vi "PC_Main3.vi"() -> ()   [LabVIEW 2017]
uses:
  <vilib>/userdefined/High Color/IMAQdx.ctl
  pc_states.ctl
  pc_data.ctl
  <vilib>/vision/Image Controls.llb/IMAQ Image.ctl
  new_coordinate.ctl
  xy_motion_graphs.ctl
  <vilib>/vision/driver/NI_Vision_Acquisition_Software.lvlib
  <vilib>/vision/NI_Vision_Development_Module.lvlib
panel:
  out "Kicker Angle":dbl caption="Numeric" format="%#.1f°"
  out "Puck Y Post":dbl
  out "Puck X Post":sgl
  out "start time":timestamp
  out "Shot Count":i16 caption="Numeric"
  out "Theta  Angle":dbl caption="Numeric" format="%#_g°"
  out "Kicker Power":dbl caption="Numeric" format="%#.1g%%"
  in  "Config Input":T1
  out "Config Output":T3
  out "Elapsed Time (s)":dbl caption="Numeric" format="%#.1p"
  out "Y Axis":dbl[][](graph) caption="Waveform Chart"
  out "X Axis":dbl[][](graph) caption="Waveform Chart"
  in  "Bounce/Straight":bool
  in  "Live Feed":bool caption="Reset"
  in  "Start":bool
  in  "Filpped":bool
  out "Live Image":T4(plugin-control)
  in  "Config":bool
  out "Snapshot Image":T4(plugin-control)
  in  "Stop":bool
  # "Table Football"
  # "UI Elements by JKI"
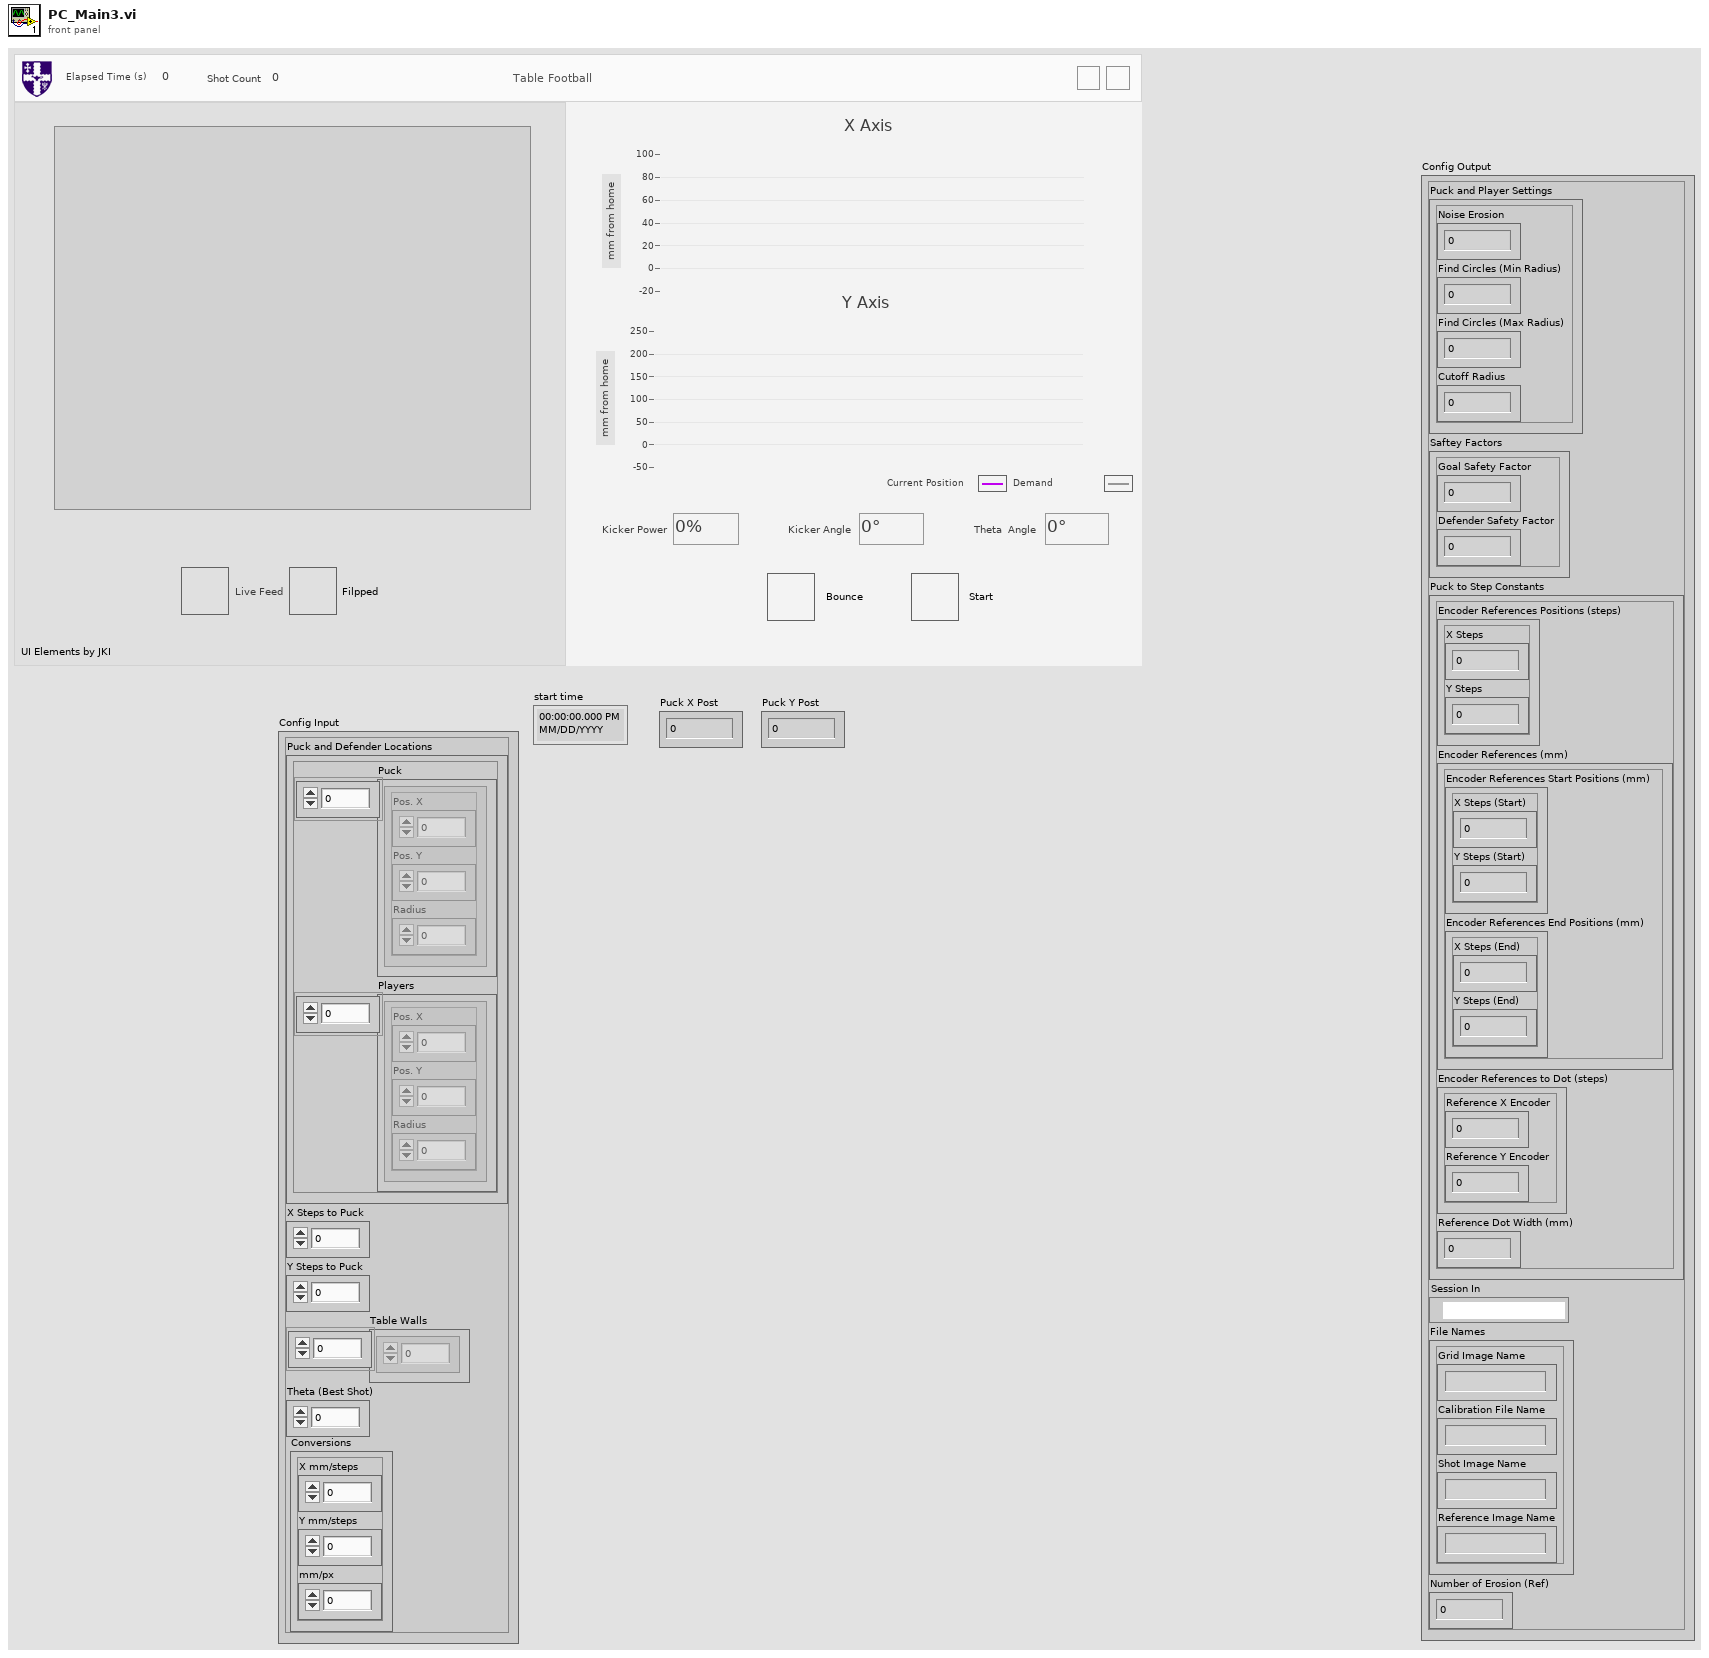
[diagram p1: front panel]
types:
  T1 = cluster{"Puck and Defender Locations":cluster{"Puck":cluster{"Pos. X":i32, "Pos. Y":i32, "Radius":i32}[], "Players":cluster{"Pos. X":i32, "Pos. Y":i32, "Radius":i32}[]}, "X Steps to Puck":dbl, "Y Steps to Puck":dbl, "Table Walls":sgl[], "Theta (Best Shot)":dbl, "Conversions":cluster{"X mm/steps":dbl, "Y mm/steps":dbl, "mm/px":dbl}}
  T2 = typedef "IMAQdx.ctl" = refnum<k21>
  T3 = cluster{"Puck and Player Settings":cluster{"Noise Erosion":i32, "Find Circles (Min Radius)":sgl, "Find Circles (Max Radius)":sgl, "Cutoff Radius  ":sgl}, "Saftey Factors":cluster{"Goal Safety Factor":dbl, "Defender Safety Factor":dbl}, "Puck to Step Constants":cluster{"Encoder References Positions (steps)":cluster{"X Steps":dbl, "Y Steps":dbl}, "Encoder References (mm)":cluster{"Encoder References Start Positions (mm)":cluster{"X Steps (Start)":dbl, "Y Steps (Start)":dbl}, "Encoder References End Positions (mm)":cluster{"X Steps (End)":dbl, "Y Steps (End)":dbl}}, "Encoder References to Dot (steps)":cluster{"Reference X Encoder":dbl, "Reference Y Encoder":dbl}, "Reference Dot Width (mm)":dbl}, "Session In":T2, "File Names":cluster{"Grid Image Name":string, "Calibration File Name":string, "Shot Image Name":string, "Reference Image Name":string}, "Number of Erosion (Ref)":i32}
  T4 = typedef "IMAQ Image.ctl" = refnum<image>
  T5 = typedef "pc_data.ctl" = cluster{"Camera Image":T4, "Reference Dimentions Out":cluster{"X":dbl, "Y":dbl, "Width":dbl}, "Table Walls":sgl[], "Player & Puck Locations":cluster{"Puck":cluster{"Pos. X":i32, "Pos. Y":i32, "Radius":i32}[], "Players":cluster{"Pos. X":i32, "Pos. Y":i32, "Radius":i32}[]}, "Theta (Best Shot)":dbl, "X Steps to Puck":dbl, "Y Steps to Puck":dbl, "Conversions":cluster{dbl, dbl, dbl}, "Shot Coordinate Template":cluster{cluster{"Straight Goal X":sgl, "Straight Goal Y":dbl}, cluster{"Bounce Wall X":dbl, "Bounce Wall Y":sgl}, cluster{"Bounce Goal X":sgl, "Bounce Goal Y":dbl}}, "Shot Power":dbl}
  T6 = typedef "Image Type" = u32
  T7 = typedef "pc_states.ctl" = cluster{enum16{"Stop", "Startup", "New Calibration Image", "Create Calibration File", "New Reference Image", "Apply Calibration (Ref)", "Find Reference Dot", "New Table Image", "Apply Calibration (Tab)", "Find Pucks, Players & Corners", "Calculate Shot Trajectories", "Calculate Puck to Steps", "Clear Best Shot Overlay", "Send Coordinates", "Update Configuration Pane", "Shot Power", "Post Shot"}, variant}
  T8 = typedef "ROI Descriptor" = cluster{"Global Rectangle":i32[], "Contours":cluster{"ID":enum32{"External", "Internal"}, "Type":u32, "Coordinates":i32[]}[]}
  T9 = enum16{"Stop", "Startup", "New Calibration Image", "Create Calibration File", "New Reference Image", "Apply Calibration (Ref)", "Find Reference Dot", "New Table Image", "Apply Calibration (Tab)", "Find Pucks, Players & Corners", "Calculate Shot Trajectories", "Calculate Puck to Steps", "Clear Best Shot Overlay", "Send Coordinates", "Update Configuration Pane", "Shot Power", "Post Shot"}
  T10 = enum8{"Enabled", "Disabled", "Disabled and Grayed Out"}
  T11 = cluster{"Goal Safety Factor":dbl, "Defender Safety Factor":dbl}
  T12 = cluster{"Noise Erosion":i32, "Find Circles (Min Radius)":sgl, "Find Circles (Max Radius)":sgl, "Cutoff Radius  ":sgl}
  T13 = cluster{"Puck":cluster{"Pos. X":i32, "Pos. Y":i32, "Radius":i32}[], "Players":cluster{"Pos. X":i32, "Pos. Y":i32, "Radius":i32}[]}
  T14 = cluster{cluster{"Straight Goal X":sgl, "Straight Goal Y":dbl}, cluster{"Bounce Wall X":dbl, "Bounce Wall Y":sgl}, cluster{"Bounce Goal X":sgl, "Bounce Goal Y":dbl}}
  T15 = cluster{"Encoder References Positions (steps)":cluster{"X Steps":dbl, "Y Steps":dbl}, "Encoder References (mm)":cluster{"Encoder References Start Positions (mm)":cluster{"X Steps (Start)":dbl, "Y Steps (Start)":dbl}, "Encoder References End Positions (mm)":cluster{"X Steps (End)":dbl, "Y Steps (End)":dbl}}, "Encoder References to Dot (steps)":cluster{"Reference X Encoder":dbl, "Reference Y Encoder":dbl}, "Reference Dot Width (mm)":dbl}
  T16 = cluster{"X Steps to Puck":dbl, "Y Steps to Puck":dbl, "Theta (Best Shot)":dbl, "Shot Power":dbl}
  T17 = cluster{"Pos. X":i32, "Pos. Y":i32, "Radius":i32}[]
  T18 = cluster{"Pos. X":i32, "Pos. Y":i32, "Radius":i32}
  T19 = typedef "xy_motion_graphs.ctl" = cluster{"Waveform Chart":dbl[][], "Waveform Chart":dbl[][]}
  T20 = cluster{"Puck and Player Settings":cluster{"Noise Erosion":i32, "Find Circles (Min Radius)":sgl, "Find Circles (Max Radius)":sgl, "Cutoff Radius  ":sgl}, "Saftey Factors":cluster{"Goal Safety Factor":dbl, "Defender Safety Factor":dbl}, "Puck to Step Constants":cluster{"Encoder References Positions (steps)":cluster{"X Steps":dbl, "Y Steps":dbl}, "Encoder References (mm)":cluster{"Encoder References Start Positions (mm)":cluster{"X Steps (Start)":dbl, "Y Steps (Start)":dbl}, "Encoder References End Positions (mm)":cluster{"X Steps (End)":dbl, "Y Steps (End)":dbl}}, "Encoder References to Dot (steps)":cluster{"Reference X Encoder":dbl, "Reference Y Encoder":dbl}, "Reference Dot Width (mm)":dbl}, "Session In":T2, "Fine Names":cluster{"Grid Image Name":string, "Calibration File Name":string, "Shot Image Name":string, "Reference Image Name":string}, "Number of Erosion (Ref)":i32}
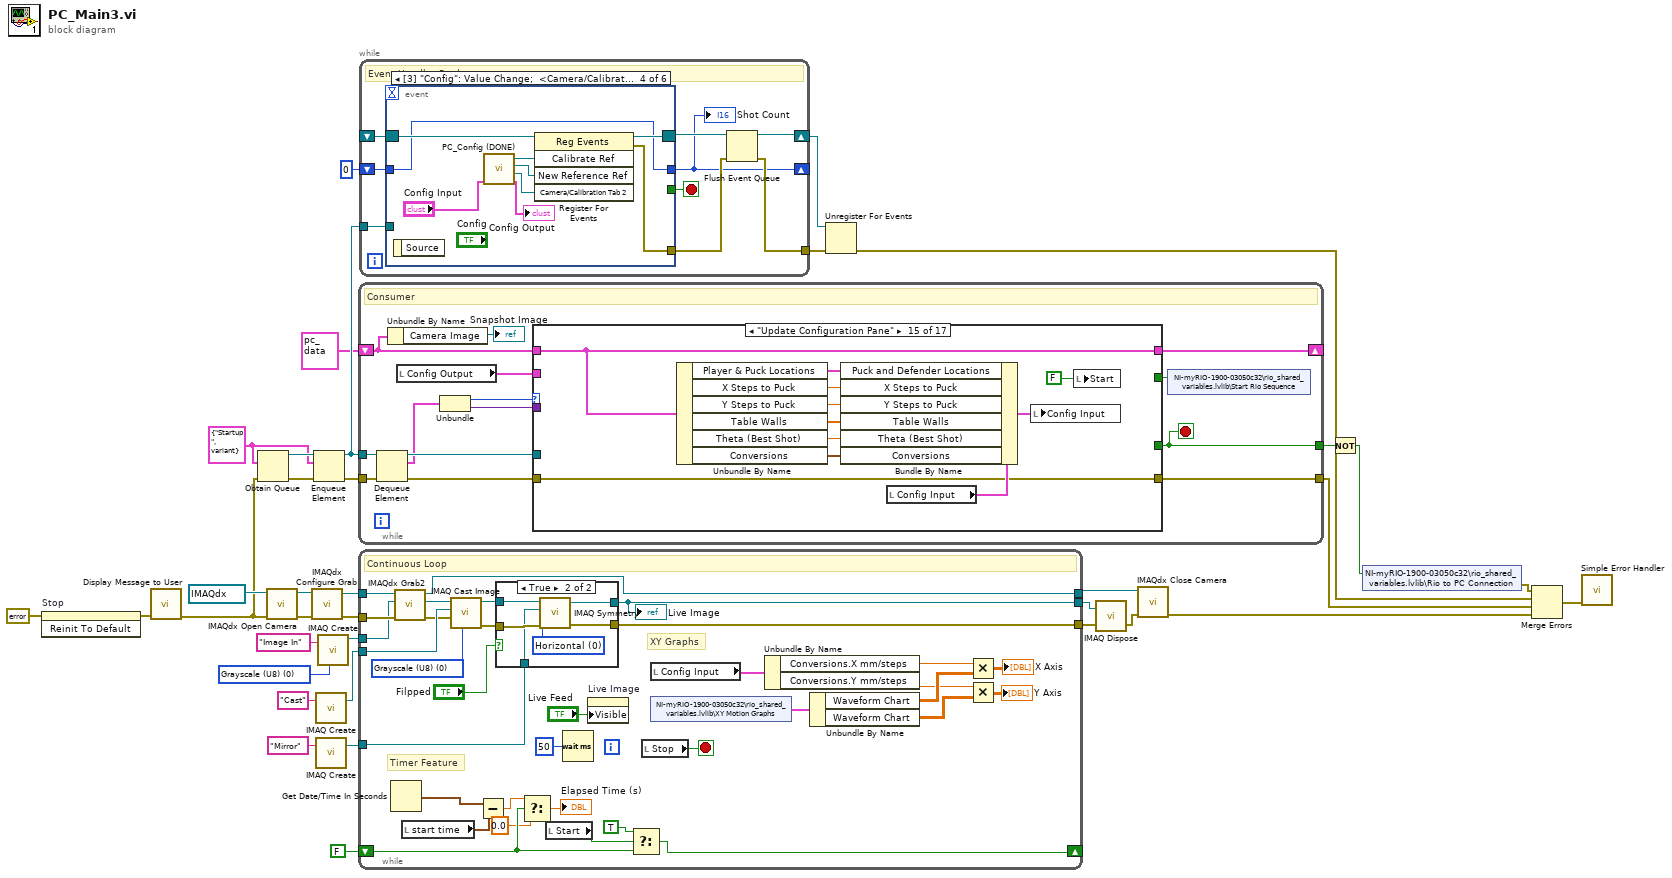
[diagram p0: block diagram]
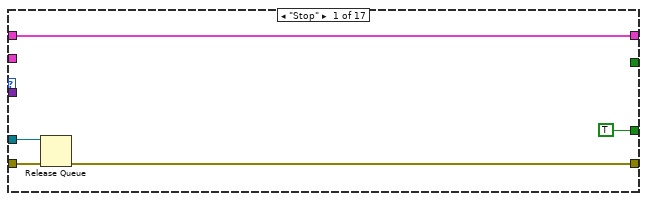
[diagram p3: hidden frame]
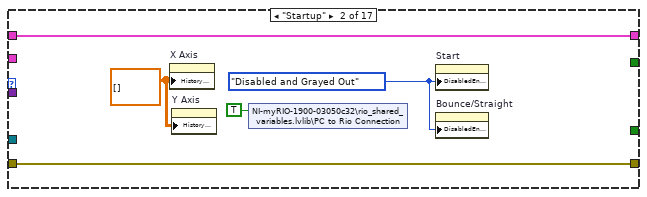
[diagram p4: hidden frame]
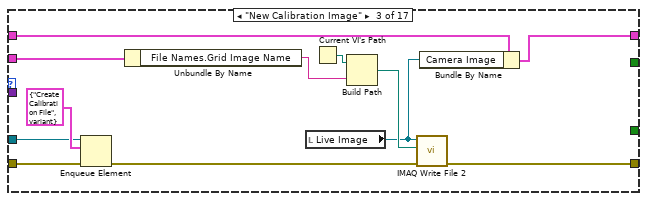
[diagram p5: hidden frame]
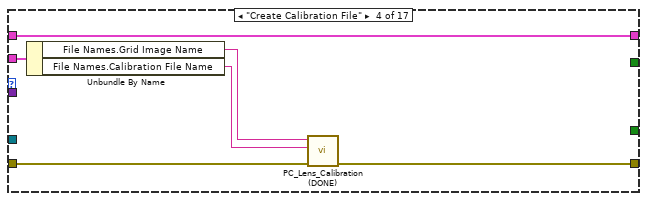
[diagram p6: hidden frame]
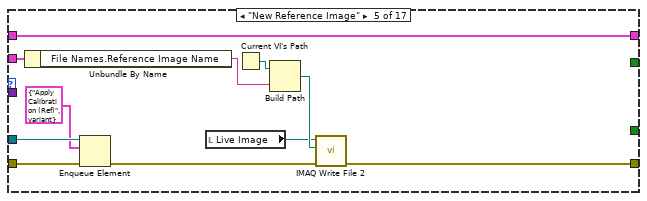
[diagram p7: hidden frame]
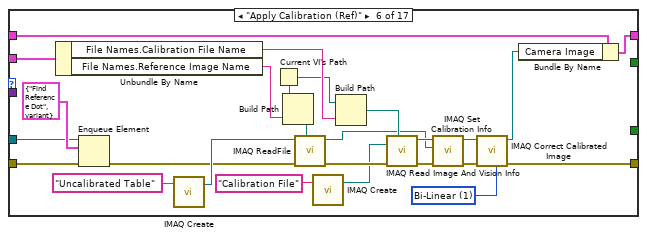
[diagram p8: hidden frame]
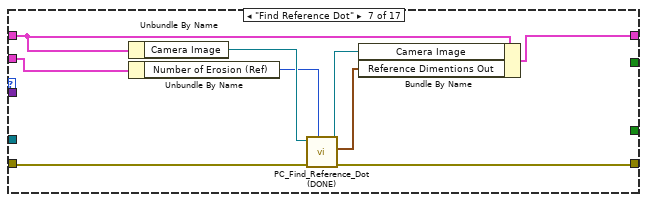
[diagram p9: hidden frame]
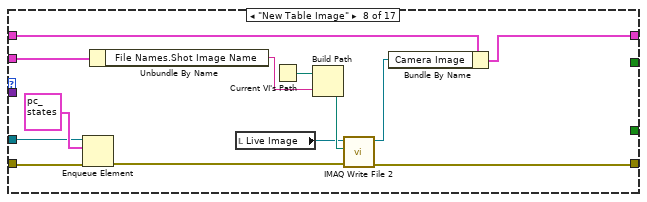
[diagram p10: hidden frame]
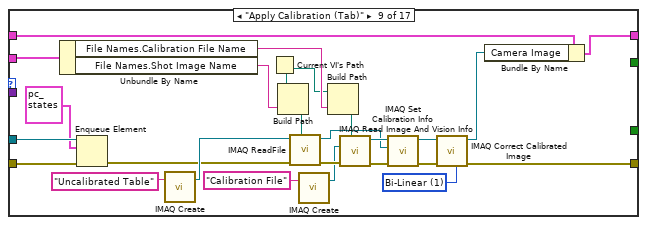
[diagram p11: hidden frame]
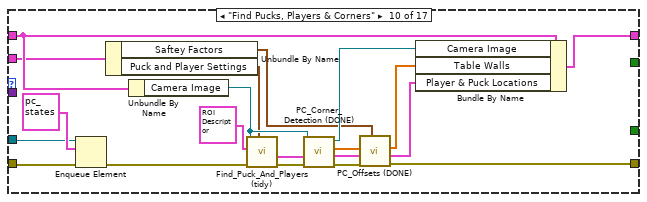
[diagram p12: hidden frame]
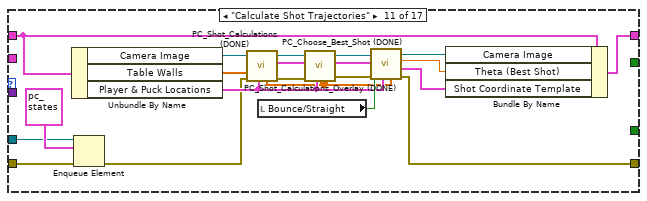
[diagram p13: hidden frame]
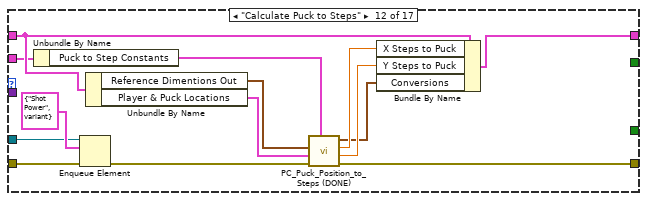
[diagram p14: hidden frame]
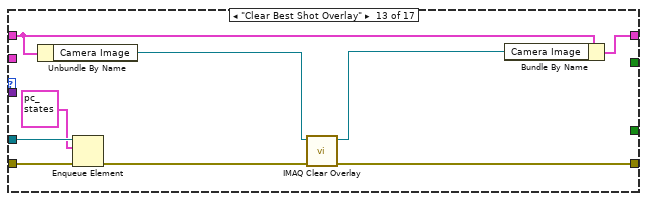
[diagram p15: hidden frame]
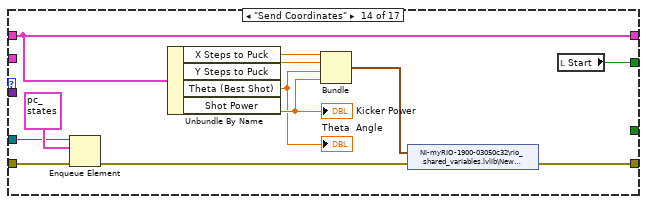
[diagram p16: hidden frame]
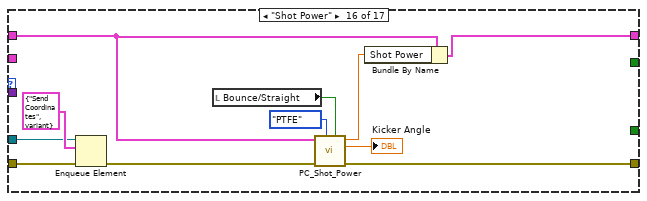
[diagram p17: hidden frame]
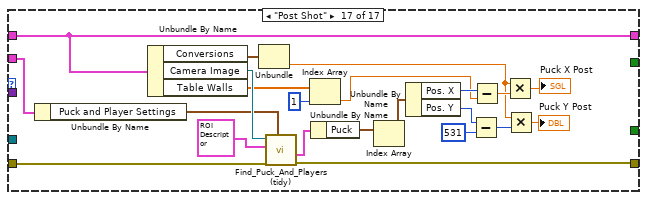
[diagram p18: hidden frame]
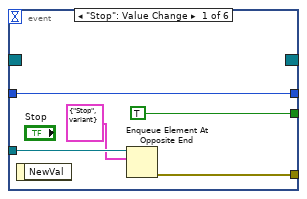
[diagram p19: hidden frame]
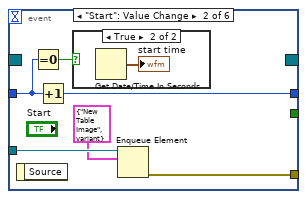
[diagram p20: hidden frame]
diagram:
  w25 = T6 0 items=["Grayscale (U8)", "Grayscale (I16)", "Grayscale (SGL)", "Complex (CSG)", "RGB (U32)", "HSL (U32)", "RGB (U64)", "Grayscale (U16)"] ("Image Type")
  w30 = T7 {enum."Startup", variant}
  n1 = invoke on="Stop" class="Bool (strict)" method="Reinit To Default"(error in=errorcluster {"status"=FALSE, "code"=0, "source"=""}) -> (error out=w1:errorcluster)  [unwired: 2 in, 2 out]
  n2 = call "Display Message to User"("error in (no error)"=w1) -> ("error out"=w2:errorcluster)  [unwired: 9 in, 1 out]
  n3 = Obtain Queue(element data type=w30, error in (no error)=w2) -> (queue out=w34:refnum<queue>, error out=w35:errorcluster)  [unwired: 3 in, 1 out]
  n4 = call <vilib>:"IMAQdx Open Camera.vi"("error in"=w2, "Session In"=T2 "cam1") -> ("error out"=w8:errorcluster, "Session Out"=w9:T2)  [unwired: 8 in]
  n5 = call <vilib>:"IMAQdx Configure Grab.vi"("error in"=w8, "Session In"=w9) -> ("error out"=w6:errorcluster, "Session Out"=w7:T2)  [unwired: 8 in]
  n6 = Enqueue Element(queue=w34, element=w30, error in (no error)=w35) -> (queue out=w32:refnum<queue>, error out=w33:errorcluster)  [unwired: 1 in, 1 out]
  n7 = call "IMAQ Create"("Image Name"="Cast") -> ("New Image"=w23:T4)  [unwired: 4 in, 1 out]
  n8 = call "IMAQ Create"("Image Name"="Mirror") -> ("New Image"=w16:T4)  [unwired: 4 in, 1 out]
  n9 = call "IMAQ Create"("Image Name"="Image In", "Image Type"=w25) -> ("New Image"=w26:T4)  [unwired: 3 in, 1 out]
  n10 = while {
    tunnel: w32 -> [w48]
    tunnel: w33 -> [w49]
    tunnel: [w50] -> w36
    tunnel: [w42] -> w22
    shift-right: [w41] -> _
    shift-left: T5 {"Camera Image"=refnum, "Reference Dimentions Out"={"X"=0.0, "Y"=0.0, "Width"=0.0}, "Table Walls"=[], "Player & Puck Locations"={"Puck"=[], "Players"=[]}, "Theta (Best Shot)"=0.0, "X Steps to Puck"=0.0, "Y Steps to Puck"=0.0, "Conversions"={0.0, 0.0, 0.0}, "Shot Coordinate Template"={{"Straight Goal X"=0.0, "Straight Goal Y"=0.0}, {"Bounce Wall X"=0.0, "Bounce Wall Y"=0.0}, {"Bounce Goal X"=0.0, "Bounce Goal Y"=0.0}}, "Shot Power"=0.0} -> [w40]
    stop <- w42 stop-if-true
    # "Consumer"
    n11 = Dequeue Element(queue=w48, error in (no error)=w49) -> (queue out=w47:refnum<queue>, element=w45:T7, error out=w46:errorcluster)  [unwired: 1 in, 1 out]
    n12 = Unbundle By Name(w40) -> ("Camera Image"=→"Snapshot Image":T4)
    n13 = local read "Config Output"() -> (w38:T3)
    n14 = Unbundle(w45) -> (w44:T9, w43:variant)
    n15 = case "Message Cases" shown="\"Update Configuration Pane\"" w44 {
      tunnel: w47 -> [w55 _ w67 _ w84 w96 _ w131 w147 w174 w184 w206 w220 w230 _ w255 _]
      tunnel: w46 -> [w52 w60 w69 w78 w85 w98 w123 w133 w148 w173 w187 w209 w221 w231 w236 w256 w276]
      tunnel: [w53 w60 w72 w77 w82 w95 w122 w132 w143 w167 w195 w214 w223 w228 w236 w253 w279] -> w50
      tunnel: [TRUE _ _ _ _ _ _ _ _ _ _ _ _ _ _ _ _] -> w42
      tunnel: w43 -> [_ _ _ _ _ _ _ _ _ _ _ _ _ _ _ _ _]
      tunnel: w40 -> [w51 w59 w65 w74 w80 w94 w119 w128 w141 w170 w193 w212 w217 w224 w246 w252 w278]
      tunnel: [w51 w59 w64 w74 w80 w93 w121 w127 w140 w169 w192 w213 w216 w224 w246 w251 w278] -> w41
      tunnel: w38 -> [_ _ w62 w73 w79 w91 w116 w125 w138 w164 _ w203 _ _ _ _ w274]
      tunnel: [_ _ _ _ _ _ _ _ _ _ _ _ _ w229 _ _ _] -> w37
      frame "Stop" {
        # "Exit - Exit the application. Since this message was sent as a priority message (i.e., it was placed at the front of the queue), any cleanup code should run here, since the loop is about to stop. Any other messages in the queue will not be handled."
        n16 = Release Queue(queue=w55, error in (no error)=w52) -> (error out=w53:errorcluster)  [unwired: 1 in, 2 out]
      }
      frame "Startup" {
        w57 = T10."Disabled and Grayed Out" ("Disabled")
        w58 = dbl[][] [] ("History Data")
        n17 = property on="X Axis" class="WFChart (strict)"("History Data"=w58) -> ()  [unwired: 2 in, 2 out]
        n18 = property on="Y Axis" class="WFChart (strict)"("History Data"=w58) -> ()  [unwired: 2 in, 2 out]
        n19 = shared-variable "NI-myRIO-1900-03050c32\\rio_shared_variables.lvlib\\PC to Rio Connection"(TRUE ("PC to Rio Connection")) -> ()  [unwired: 1 in, 1 out]
        n20 = property on="Start" class="Bool (strict)"("DisabledEnum"=w57) -> ()  [unwired: 2 in, 2 out]
        n21 = property on="Bounce/Straight" class="Bool (strict)"("DisabledEnum"=w57) -> ()  [unwired: 2 in, 2 out]
      }
      frame "New Calibration Image" {
        n22 = Enqueue Element(queue=w67, element=T7 {enum."Create Calibration File", variant}, error in (no error)=w69) -> (error out=w66:errorcluster)  [unwired: 1 in, 2 out]
        n23 = Unbundle By Name(w62) -> ("File Names.Grid Image Name"=w61:string)
        n24 = local read "Live Image"() -> (w63:T4)
        n25 = Current VI's Path() -> (path=w70:path)
        n26 = Build Path(base path=w70, name or relative path=w61) -> (appended path=w71:path)
        n27 = call-poly "IMAQ Write File 2"("error in (no error)"=w66, "File Path"=w71, "Image"=w63) -> ("error out"=w72:errorcluster)  [unwired: 7 in, 1 out]
        n28 = Bundle By Name(cluster=w65, "Camera Image"=w63) -> (w64:T5)
      }
      frame "Create Calibration File" {
        n29 = Unbundle By Name(w73) -> ("File Names.Grid Image Name"=w76:string, "File Names.Calibration File Name"=w75:string)
        n30 = call "PC_Lens_Calibration (DONE).vi"("Error In"=w78, "Calibration File Name"=w75, "Grid Image Name"=w76) -> ("Error Out"=w77:errorcluster)  [unwired: 8 in]
      }
      frame "New Reference Image" {
        n31 = Unbundle By Name(w79) -> ("File Names.Reference Image Name"=w87:string)
        n32 = Enqueue Element(queue=w84, element=T7 {enum."Apply Calibration (Ref)", variant}, error in (no error)=w85) -> (error out=w86:errorcluster)  [unwired: 1 in, 2 out]
        n33 = local read "Live Image"() -> (w83:T4)
        n34 = Current VI's Path() -> (path=w88:path)
        n35 = Build Path(base path=w88, name or relative path=w87) -> (appended path=w89:path)
        n36 = call-poly "IMAQ Write File 2"("error in (no error)"=w86, "File Path"=w89, "Image"=w83) -> ("error out"=w82:errorcluster)  [unwired: 7 in, 1 out]
      }
      frame "Apply Calibration (Ref)" {
        w100 = u32 1 items=["Zero Order", "Bi-Linear", "Quadratic", "Cubic Spline"] ("Interpolation Type")
        n37 = Unbundle By Name(w91) -> ("File Names.Calibration File Name"=w103:string, "File Names.Reference Image Name"=w104:string)
        n38 = Enqueue Element(queue=w96, element=T7 {enum."Find Reference Dot", variant}, error in (no error)=w98) -> (error out=w97:errorcluster)  [unwired: 1 in, 2 out]
        n39 = call "IMAQ Create"("Image Name"="Uncalibrated Table") -> ("New Image"=w107:T4)  [unwired: 4 in, 1 out]
        n40 = Current VI's Path() -> (path=w90:path)
        n41 = Build Path(base path=w90, name or relative path=w104) -> (appended path=w113:path)
        n42 = call "IMAQ ReadFile"("File Path"=w113, "error in (no error)"=w97, "Image"=w107) -> ("error out"=w114:errorcluster, "Image Out"=w105:T4)  [unwired: 4 in, 3 out]
        n43 = call "IMAQ Create"("Image Name"="Calibration File") -> ("New Image"=w108:T4)  [unwired: 4 in, 1 out]
        n44 = Build Path(base path=w90, name or relative path=w103) -> (appended path=w112:path)
        n45 = call "IMAQ Read Image And Vision Info"("File Path"=w112, "error in (no error)"=w114, "Image"=w108) -> ("error out"=w110:errorcluster, "Image Out"=w106:T4)  [unwired: 6 in, 1 out]
        n46 = call "IMAQ Set Calibration Info"("error in (no error)"=w110, "Image Dst"=w105, "Image Src"=w106) -> ("error out"=w111:errorcluster, "Calibrated Image"=w109:T4)  [unwired: 7 in]
        n47 = call "IMAQ Correct Calibrated Image"("Interpolation Type"=w100, "error in (no error)"=w111, "Image Src"=w109) -> ("error out"=w95:errorcluster, "Corrected Image"=w92:T4)  [unwired: 7 in]
        n48 = Bundle By Name(cluster=w94, "Camera Image"=w92) -> (w93:T5)
      }
      frame "Find Reference Dot" {
        n49 = Unbundle By Name(w119) -> ("Camera Image"=w118:T4)
        n50 = Unbundle By Name(w116) -> ("Number of Erosion (Ref)"=w115:i32)
        n51 = call "PC_Find_Reference_Dot (DONE).vi"("Number of Erosion in"=w115, "Error In"=w123, "Image In"=w118) -> ("Error Out"=w122:errorcluster, "Reference Dimentions Out"=w120:cluster{"X":dbl, "Y":dbl, "Width":dbl}, "Image Out"=w117:T4)  [unwired: 6 in]
        n52 = Bundle By Name(cluster=w119, "Camera Image"=w117, "Reference Dimentions Out"=w120) -> (w121:T5)
      }
      frame "New Table Image" {
        n53 = Enqueue Element(queue=w131, element=T7 {enum."Apply Calibration (Tab)", variant}, error in (no error)=w133) -> (error out=w129:errorcluster)  [unwired: 1 in, 2 out]
        n54 = Unbundle By Name(w125) -> ("File Names.Shot Image Name"=w124:string)
        n55 = local read "Live Image"() -> (w130:T4)
        n56 = Current VI's Path() -> (path=w135:path)
        n57 = Build Path(base path=w135, name or relative path=w124) -> (appended path=w136:path)
        n58 = call-poly "IMAQ Write File 2"("error in (no error)"=w129, "File Path"=w136, "Image"=w130) -> ("error out"=w132:errorcluster, "Image Out (duplicate)"=w126:T4)  [unwired: 7 in]
        n59 = Bundle By Name(cluster=w128, "Camera Image"=w126) -> (w127:T5)
      }
      frame "Apply Calibration (Tab)" {
        w157 = u32 1 items=["Zero Order", "Bi-Linear", "Quadratic", "Cubic Spline"] ("Interpolation Type")
        n60 = Unbundle By Name(w138) -> ("File Names.Calibration File Name"=w144:string, "File Names.Shot Image Name"=w145:string)
        n61 = Enqueue Element(queue=w147, element=T7 {enum."Find Pucks, Players & Corners", variant}, error in (no error)=w148) -> (error out=w146:errorcluster)  [unwired: 1 in, 2 out]
        n62 = call "IMAQ Create"("Image Name"="Uncalibrated Table") -> ("New Image"=w153:T4)  [unwired: 4 in, 1 out]
        n63 = Current VI's Path() -> (path=w137:path)
        n64 = Build Path(base path=w137, name or relative path=w145) -> (appended path=w160:path)
        n65 = call "IMAQ ReadFile"("File Path"=w160, "error in (no error)"=w146, "Image"=w153) -> ("error out"=w161:errorcluster, "Image Out"=w149:T4)  [unwired: 4 in, 3 out]
        n66 = call "IMAQ Create"("Image Name"="Calibration File") -> ("New Image"=w154:T4)  [unwired: 4 in, 1 out]
        n67 = Build Path(base path=w137, name or relative path=w144) -> (appended path=w159:path)
        n68 = call "IMAQ Read Image And Vision Info"("File Path"=w159, "error in (no error)"=w161, "Image"=w154) -> ("error out"=w156:errorcluster, "Image Out"=w150:T4)  [unwired: 6 in, 1 out]
        n69 = call "IMAQ Set Calibration Info"("error in (no error)"=w156, "Image Dst"=w149, "Image Src"=w150) -> ("error out"=w158:errorcluster, "Calibrated Image"=w155:T4)  [unwired: 7 in]
        n70 = call "IMAQ Correct Calibrated Image"("Interpolation Type"=w157, "error in (no error)"=w158, "Image Src"=w155) -> ("error out"=w143:errorcluster, "Corrected Image"=w139:T4)  [unwired: 7 in]
        n71 = Bundle By Name(cluster=w141, "Camera Image"=w139) -> (w140:T5)
      }
      frame "Find Pucks, Players & Corners" {
        n72 = Enqueue Element(queue=w174, element=T7 {enum."Calculate Shot Trajectories", variant}, error in (no error)=w173) -> (error out=w172:errorcluster)  [unwired: 1 in, 2 out]
        n73 = Unbundle By Name(w164) -> ("Saftey Factors"=w163:T11, "Puck and Player Settings"=w162:T12)
        n74 = Unbundle By Name(w170) -> ("Camera Image"=w171:T4)
        n75 = call "Find_Puck_And_Players (tidy).vi"("Puck and Player Settings"=w162, "Error In"=w172, "ROI Descriptor (Tab) in"=T8 {"Global Rectangle"=[156, 32, 1271, 1029], "Contours"=[{"ID"=enum."External", "Type"=12, "Coordinates"=[156, 32, 1271, 1029, 0]}]} ("ROI Descriptor (Tab)"), "Image In"=w171) -> ("Error Out"=w179:errorcluster, "Puck and Player Position"=w176:T13)  [unwired: 6 in]
        n76 = call "PC_Corner_Detection (DONE).vi"("Error In"=w179, "Puck and Player Position"=w176, "Image In"=w171) -> ("Error Out"=w180:errorcluster, "Puck and Player Position (Through)"=w177:T13, "Table Walls"=w181:sgl[], "Image Out"=w168:T4)  [unwired: 5 in]
        n77 = call "PC_Offsets (DONE).vi"("Saftey Factors"=w163, "Error In"=w180, "Puck and Defender Inputs"=w177, "Table Walls Input"=w181) -> ("Error Out"=w167:errorcluster, "Puck and Defender Output"=w165:T13, "Table Walls Output"=w166:sgl[])  [unwired: 5 in]
        n78 = Bundle By Name(cluster=w170, "Camera Image"=w168, "Table Walls"=w166, "Player & Puck Locations"=w165) -> (w169:T5)
      }
      frame "Calculate Shot Trajectories" {
        n79 = Unbundle By Name(w193) -> ("Camera Image"=w194:T4, "Table Walls"=w188:sgl[], "Player & Puck Locations"=w189:T13)
        n80 = Enqueue Element(queue=w184, element=T7 {enum."Calculate Puck to Steps", variant}, error in (no error)=w187) -> (error out=w186:errorcluster)  [unwired: 1 in, 2 out]
        n81 = call "PC_Shot_Calculations (DONE).vi"("Table Walls Input"=w188, "Player and Puck Input"=w189, "Error In"=w186) -> ("Error Out"=w196:errorcluster, "Shot Outputs"=w199:cluster{"Bounce":dbl[][], "Straight":dbl[][]})  [unwired: 7 in]
        n82 = local read "Bounce/Straight"() -> (w190:bool)
        n83 = call "PC_Shot_Calculations_Overlay (DONE).vi"("Table Walls Input"=w188, "Player and Puck Input"=w189, "Error  In"=w196, "Shot Inputs"=w199, "Image In"=w194) -> ("Error Out"=w197:errorcluster, "Shot Outputs (Pass Through)"=w200:cluster{"Bounce":dbl[][], "Straight":dbl[][]}, "Image Out"=w198:T4)  [unwired: 4 in]
        n84 = call "PC_Choose_Best_Shot (DONE).vi"("Table Walls Inputs"=w188, "Straight/Bounce"=w190, "Puck and Players In"=w189, "Error In"=w197, "Shot Inputs"=w200, "Image In"=w198) -> ("Error Out"=w195:errorcluster, "Shot Coordinate"=w182:T14, "Best Shot Theta"=w183:dbl, "Image Out"=w191:T4)  [unwired: 2 in]
        n85 = Bundle By Name(cluster=w193, "Camera Image"=w191, "Theta (Best Shot)"=w183, "Shot Coordinate Template"=w182) -> (w192:T5)
      }
      frame "Calculate Puck to Steps" {
        n86 = Unbundle By Name(w203) -> ("Puck to Step Constants"=w202:T15)
        n87 = Enqueue Element(queue=w206, element=T7 {enum."Shot Power", variant}, error in (no error)=w209) -> (error out=w208:errorcluster)  [unwired: 1 in, 2 out]
        n88 = Unbundle By Name(w212) -> ("Reference Dimentions Out"=w211:cluster{"X":dbl, "Y":dbl, "Width":dbl}, "Player & Puck Locations"=w210:T13)
        n89 = call "PC_Puck_Position_to_Steps (DONE).vi"("Puck to Step Constants"=w202, "Error In"=w208, "Puck and Defender Output (pixels)"=w210, "Reference Dot Dimentions In (pixels)"=w211) -> ("Error Out"=w214:errorcluster, "Y Steps to Puck"=w204:dbl, "X Steps to Puck"=w205:dbl, "Conversions"=w201:cluster{dbl, dbl, dbl})  [unwired: 3 in]
        n90 = Bundle By Name(cluster=w212, "X Steps to Puck"=w205, "Y Steps to Puck"=w204, "Conversions"=w201) -> (w213:T5)
      }
      frame "Clear Best Shot Overlay" {
        n91 = Unbundle By Name(w217) -> ("Camera Image"=w218:T4)
        n92 = Enqueue Element(queue=w220, element=T7 {enum."Calculate Shot Trajectories", variant}, error in (no error)=w221) -> (error out=w222:errorcluster)  [unwired: 1 in, 2 out]
        n93 = call "IMAQ Clear Overlay"("error in (no error)"=w222, "Image"=w218) -> ("error out"=w223:errorcluster, "Image Out"=w215:T4)  [unwired: 8 in]
        n94 = Bundle By Name(cluster=w217, "Camera Image"=w215) -> (w216:T5)
      }
      frame "Send Coordinates" {
        n95 = Enqueue Element(queue=w230, element=T7 {enum."Update Configuration Pane", variant}, error in (no error)=w231) -> (error out=w232:errorcluster)  [unwired: 1 in, 2 out]
        n96 = Unbundle By Name(w224) -> ("X Steps to Puck"=w235:dbl, "Y Steps to Puck"=w234:dbl, "Theta (Best Shot)"=w225:dbl, "Shot Power"=w226:dbl)
        "Kicker Power" <- w226
        "Theta  Angle" <- w225
        n97 = Bundle("X Steps to Puck"=w235, "Y Steps to Puck"=w234, "Theta (Best Shot)"=w225, "Shot Power"=w226) -> (w227:T16)  [unwired: 1 in]
        n98 = shared-variable "NI-myRIO-1900-03050c32\\rio_shared_variables.lvlib\\New Coordinate"(w227, error in=w232) -> (error out=w228:errorcluster)
        n99 = local read "Start"() -> (w229:bool)
      }
      frame "Update Configuration Pane" {
        n100 = Unbundle By Name(w246) -> ("Player & Puck Locations"=w245:T13, "X Steps to Puck"=w244:dbl, "Y Steps to Puck"=w243:dbl, "Table Walls"=w242:sgl[], "Theta (Best Shot)"=w241:dbl, "Conversions"=w237:cluster{dbl, dbl, dbl})
        n101 = local read "Config Input"() -> (w238:T1)
        n102 = Bundle By Name(cluster=w238, "Puck and Defender Locations"=w245, "X Steps to Puck"=w244, "Y Steps to Puck"=w243, "Table Walls"=w242, "Theta (Best Shot)"=w241, "Conversions"=w237) -> (w239:T1)
        n103 = local write "Config Input"(w239) -> ()
        n104 = local write "Start"(FALSE ("Start")) -> ()
      }
      frame "Shot Power" {
        n105 = Enqueue Element(queue=w255, element=T7 {enum."Send Coordinates", variant}, error in (no error)=w256) -> (error out=w254:errorcluster)  [unwired: 1 in, 2 out]
        n106 = local read "Bounce/Straight"() -> (w249:bool)
        n107 = call "PC_Shot_Power.vi"("Bounce T/F?"=w249, "Puck Selection"=enum32{"PTFE", "Nylon"}."PTFE", "Error In"=w254, "PC Data"=w252) -> ("Error Out"=w253:errorcluster, "Kicker angle"=→"Kicker Angle":dbl, "Power %"=w248:dbl)  [unwired: 5 in]
        n108 = Bundle By Name(cluster=w252, "Shot Power"=w248) -> (w251:T5)
      }
      frame "Post Shot" {
        n109 = Unbundle By Name(w274) -> ("Puck and Player Settings"=w273:T12)
        n110 = Unbundle By Name(w278) -> ("Conversions"=w259:cluster{dbl, dbl, dbl}, "Camera Image"=w277:T4, "Table Walls"=w272:sgl[])
        n111 = Unbundle(w259) -> (w258:dbl)  [unwired: 2 out]
        n112 = call "Find_Puck_And_Players (tidy).vi"("Puck and Player Settings"=w273, "Error In"=w276, "ROI Descriptor (Tab) in"=T8 {"Global Rectangle"=[921, 77, 1261, 985], "Contours"=[{"ID"=enum."External", "Type"=12, "Coordinates"=[921, 77, 1261, 985, 0]}]} ("ROI Descriptor"), "Image In"=w277) -> ("Error Out"=w279:errorcluster, "Puck and Player Position"=w270:T13)  [unwired: 6 in]
        n113 = Index Array(array=w272, index=1) -> (element=w266:sgl)
        n114 = Unbundle By Name(w270) -> ("Puck"=w269:T17)
        n115 = Index Array(array=w269) -> (element=w268:T18)  [unwired: 1 in]
        n116 = Unbundle By Name(w268) -> ("Pos. X"=w267:i32, "Pos. Y"=w264:i32)
        n117 = Subtract(x=w264, y=531) -> (x-y=w262:i32)
        n118 = Subtract(x=w267, y=w266) -> (x-y=w265:sgl)
        n119 = Multiply(x=w258, y=w265) -> (x*y=→"Puck X Post":dbl)
        n120 = Multiply(x=w258, y=w262) -> (x*y=→"Puck Y Post":dbl)
      }
    }
    n121 = shared-variable "NI-myRIO-1900-03050c32\\rio_shared_variables.lvlib\\Start Rio Sequence"(w37) -> ()  [unwired: 1 in, 1 out]
  }
  n122 = while {
    tunnel: w7 -> [w311]
    tunnel: w6 -> [w310]
    tunnel: [w312] -> w27
    tunnel: w26 -> [w309]
    tunnel: w23 -> [w307]
    tunnel: [w301] -> w18
    tunnel: [w299] -> w19
    tunnel: w16 -> [w302]
    shift-right: [w288] -> _
    shift-left: FALSE ("Start") -> [w282]
    stop <- w313 stop-if-true
    w305 = T6 0 items=["Grayscale (U8)", "Grayscale (I16)", "Grayscale (SGL)", "Complex (CSG)", "RGB (U32)", "HSL (U32)", "RGB (U64)", "Grayscale (U16)"] ("Image Type")
    # "XY Graphs"
    # "Timer Feature"
    # "Continuous Loop"
    n123 = Get Date/Time In Seconds() -> (seconds since 1Jan1904=w284:timestamp)
    n124 = call <vilib>:"IMAQdx Grab2.vi"("error in"=w310, "Image In"=w309, "Session In"=w311) -> ("error out"=w306:errorcluster, "Image Out"=w308:T4, "Session Out"=w312:T2)  [unwired: 5 in, 1 out]
    n125 = local read "start time"() -> (w285:timestamp)
    n126 = call "IMAQ Cast Image"("Image Type"=w305, "error in (no error)"=w306, "Image Dst"=w307, "Image Src"=w308) -> ("error out"=w303:errorcluster, "Image Dst Out"=w304:T4)  [unwired: 6 in]
    n127 = Subtract(x=w284, y=w285) -> (x-y=w281:dbl)
    n128 = case shown="True" "Filpped" {
      tunnel: w304 -> [w314 w321]
      tunnel: w303 -> [w315 w320]
      tunnel: w302 -> [_ w319]
      tunnel: [w314 w318] -> w299
      tunnel: [w315 w317] -> w301
      frame False {
      }
      frame True {
        w316 = u32 0 items=["Horizontal", "Vertical", "Central", "1st Diagonal", "2nd Diagonal"] ("Type of Symmetry")
        n129 = call "IMAQ Symmetry"("error in (no error)"=w320, "Type of Symmetry"=w316, "Image Dst"=w319, "Image Src"=w321) -> ("error out"=w317:errorcluster, "Image Dst Out"=w318:T4)  [unwired: 1 in]
      }
    }
    "Live Image" <- w299
    n130 = Select(t=w281, s=w282, f=0.0) -> (s? t:f=→"Elapsed Time (s)":dbl)
    n131 = local read "Start"() -> (w287:bool)
    n132 = Wait (ms)(milliseconds to wait=u32 50) -> ()  [unwired: 1 out]
    n133 = property on="Live Image" class="ImageControl"("Visible"="Live Feed") -> ()  [unwired: 2 in, 2 out]
    n134 = Select(t=TRUE ("Start"), s=w287, f=w282) -> (s? t:f=w288:bool)
    n135 = local read "Stop"() -> (w313:bool)
    n136 = local read "Config Input"() -> (w292:T1)
    n137 = shared-variable "NI-myRIO-1900-03050c32\\rio_shared_variables.lvlib\\XY Motion Graphs"() -> (w297:T19)  [unwired: 1 in, 1 out]
    n138 = Unbundle By Name(w292) -> ("Conversions.X mm/steps"=w291:dbl, "Conversions.Y mm/steps"=w289:dbl)
    n139 = Unbundle By Name(w297) -> ("Waveform Chart"=w294:dbl[][], "Waveform Chart"=w296:dbl[][])
    n140 = Multiply(x=w291, y=w294) -> (x*y=→"X Axis":dbl[][])
    n141 = Multiply(x=w289, y=w296) -> (x*y=→"Y Axis":dbl[][])
  }
  n142 = while {
    tunnel: w32 -> [w330]
    tunnel: [w324] -> w11
    shift-right: [w326] -> w13
    shift-left: _ -> [w328]
    shift-right: [w322] -> _
    shift-left: i16 0 ("Shot Count") -> [w323]
    stop <- w329 stop-if-true
    # "Event Handler Producer"
    n143 = event shown="[3] \"Config\": Value Change;  <Camera/Calibration Tab 2>: Value Change" {
      selector: w328 -> [_ _ _ w350 _ _]
      dyn-events: [_ _ _ w355 _ _] -> w327
      timeout: _ -> [_ _ _ _ _ _]
      tunnel: [TRUE _ _ _ _ _] -> w329
      tunnel: w330 -> [w335 w340 w344 _ w358 w364]
      tunnel: [w334 w341 w345 w349 w359 w365] -> w325
      tunnel: w323 -> [w331 w336 w343 w347 w356 w361]
      tunnel: [w331 w338 w343 w347 w356 w361] -> w322
      event "Stop": Value Change {
        # "Enqueue an \"Exit\" message. Note that the Enqueue Element At Opposite End function is used to place this priority \"Exit\" message at the front of the queue ahead of all other messages."
        n144 = event-data() -> ()  [unwired: 1 in, 1 out]
        n145 = Enqueue Element At Opposite End(queue=w335, element=T7 {enum."Stop", variant}) -> (error out=w334:errorcluster)  [unwired: 2 in, 2 out]
      }
      event "Start": Value Change {
        n146 = event-data() -> ()  [unwired: 1 in, 1 out]
        n147 = Equal To 0?(x=w336) -> (x = 0?=w337:bool)
        n148 = Increment(x=w336) -> (x+1=w338:i16)
        n149 = case shown="True" w337 {
          frame False {
          }
          frame True {
            n150 = Get Date/Time In Seconds() -> (seconds since 1Jan1904=→"start time":timestamp)
          }
        }
        n151 = Enqueue Element(queue=w340, element=T7 {enum."New Table Image", variant}) -> (error out=w341:errorcluster)  [unwired: 2 in, 2 out]
      }
      event "Bounce/Straight": Value Change {
        n152 = event-data() -> ()  [unwired: 1 in, 1 out]
        n153 = Enqueue Element(queue=w344, element=T7 {enum."New Table Image", variant}) -> (error out=w345:errorcluster)  [unwired: 2 in, 2 out]
      }
      event "Config": Value Change {
        n154 = event-data() -> ()  [unwired: 1 in, 1 out]
        n155 = call "PC_Config (DONE).vi"("Config Input"="Config Input") -> ("Config Output"=→"Config Output":T20, "Camera/Calibration Tab 2"=w351:refnum<vi>, "New Reference Ref"=w353:refnum<vi>, "Calibrate Ref"=w352:refnum<vi>)  [unwired: 3 in]
        n156 = register-events(reference=w350, w352, w353, w351) -> (reference out=w355:refnum<event-registration>, error out=w349:errorcluster)  [unwired: 1 in]
      }
      event Value Change {
        w357 = T10."Enabled" ("Disabled")
        n157 = event-data() -> ()  [unwired: 1 in, 1 out]
        n158 = Enqueue Element(queue=w358, element=T7 {enum."Create Calibration File", variant}) -> (error out=w359:errorcluster)  [unwired: 2 in, 2 out]
        n159 = property on="Start" class="Bool (strict)"("DisabledEnum"=w357) -> ()  [unwired: 2 in, 2 out]
        n160 = property on="Bounce/Straight" class="Bool (strict)"("DisabledEnum"=w357) -> ()  [unwired: 2 in, 2 out]
      }
      event Value Change {
        w362 = T10."Enabled" ("Disabled")
        n161 = event-data() -> ()  [unwired: 1 in, 1 out]
        n162 = Enqueue Element(queue=w364, element=T7 {enum."Apply Calibration (Ref)", variant}) -> (error out=w365:errorcluster)  [unwired: 2 in, 2 out]
        n163 = property on="Start" class="Bool (strict)"("DisabledEnum"=w362) -> ()  [unwired: 2 in, 2 out]
        n164 = property on="Bounce/Straight" class="Bool (strict)"("DisabledEnum"=w362) -> ()  [unwired: 2 in, 2 out]
      }
    }
    "Shot Count" <- w322
    n165 = Flush Event Queue(0:w327, 3:w325) -> (8:w326:refnum<event-registration>, 11:w324:errorcluster)  [unwired: 4 in, 1 out]
  }
  n166 = Unregister For Events(event registration refnum=w13, error in=w11) -> (error out=w12:errorcluster)
  n167 = call "IMAQ Dispose"("Image"=w19, "error in (no error)"=w18) -> ("error out"=w17:errorcluster)  [unwired: 4 in]
  n168 = call <vilib>:"IMAQdx Close Camera.vi"("error in"=w17, "Session In"=w27) -> ("error out"=w29:errorcluster)  [unwired: 9 in]
  n169 = Not(x=w22) -> (.not. x?=w21:bool)
  n170 = shared-variable "NI-myRIO-1900-03050c32\\rio_shared_variables.lvlib\\Rio to PC Connection"(w21) -> (error out=w20:errorcluster)  [unwired: 1 in]
  n171 = Merge Errors(w20, w12, w36, w29) -> (w31:errorcluster)
  n172 = call <vilib>:"Simple Error Handler.vi"("error in (no error)"=w31) -> ()  [unwired: 4 in, 5 out]
